vi "Exit Initialize (User).vi"(8 "error in":errorcluster, 11 "Node in":refnum<class "AMS Climate Chamber Template.lvclass">) -> (0 "error out":errorcluster, 3 "Node out":refnum<class "AMS Climate Chamber Template.lvclass">)   [LabVIEW 2023, in "AMS Climate Chamber Template.lvlib" / "AMS Climate Chamber Template.lvclass"]
uses:
  AMS Climate Chamber Template.lvclass
  C:/Program Files/National Instruments/LabVIEW 2024/vi.lib/ADAS Replay HIL/Template Node/Plugin/Template Node/Template Node.lvclass
  <vilib>/ADAS Replay HIL/Template Node/Plugin/Template Node/Template Node.lvclass/Template Node.ctl
  C:/Program Files/National Instruments/AMS plugin/Capabilities/Capabilities/Utilities/Utilities.lvlib
  <vilib>/ADAS Replay HIL/Template Node/Plugin/Template Node/Template Node.lvclass
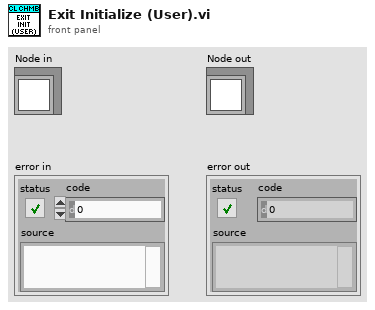
[diagram p1: front panel]
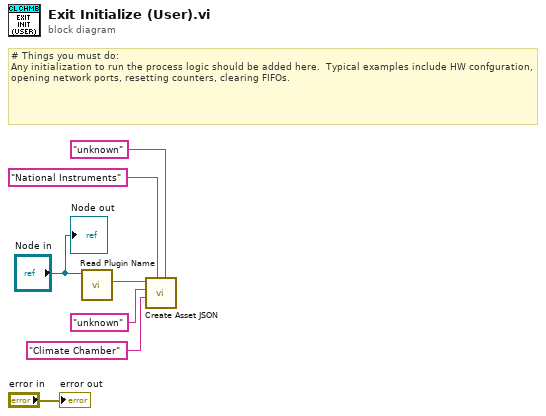
[diagram p0: block diagram]
diagram:
  # "# Things you must do:\nAny initialization to run the process logic should be added here.  Typical examples include HW confguration, opening network ports, resetting counters, clearing FIFOs."
  n1 = call <vilib>:"Read Plugin Name.vi"("Template Node in"="Node in") -> ("Plugin Name"=w6:string)  [unwired: 8 in, 2 out]
  n2 = call "Create Asset JSON.vi"("firmwareVersion"="unknown", "vendorName"="National Instruments", "modelName"="Climate Chamber", "serialNumber"="unknown", "pluginName"=w6) -> ()  [unwired: 5 in, 2 out]
  "Node out" <- "Node in"
  "error out" <- "error in"
